vi "Configure.vi"(8 "error in (no error)":errorcluster, 11 "focus in":refnum<class "focus.lvclass">) -> (0 "error out":errorcluster, 2 "cancelled?":bool, 3 "focus out":refnum<class "focus.lvclass">)   [LabVIEW 2012, in "focus.lvclass"]
doc: "The configure method configures the details for the RabbitMQ connection, the observers and the mapping script.\n\nIn the derived class, make a call to the parent for setting these parameters."
uses:
  focus.lvclass
  port_focus.ctl
  baud_rate_focus.ctl
  connection_type_focus.ctl
  <vilib>/Utility/miscctls.llb/LVPointTypeDef.ctl
  focus.lvclass/focus.ctl
  <vilib>/Distrio/Murmex/Murmex/Murmex.lvclass
panel:
  in  "button::ok":bool
  in  "button::configure murmex":bool
  in  "button::cancel":bool
  in  "Tab Control":enum32{"COM ", "Debug"}(tab)
  in  "Port":T1 items=["COM1", "COM2", "COM3", "COM4", "COM5", "COM6", "COM7", "COM8", "COM9", "COM10", "COM11", "COM12", "COM13", "COM14", "COM15", "COM16", "COM17", "COM18", "COM19", "COM20", "COM21", "COM22", "COM23", "COM24", "COM25", "COM26", "COM27", "COM28", "COM29", "COM30"]
  in  "Baudrate":T2=3 items=["9600", "14400", "19200", "38400", "57600", "115200"]
  in  "update frequency":dbl[unit]
  in  "soft limit min":dbl
  in  "soft limit max":dbl
  in  "S/N Master controller":string
  in  "Interface":T3=enum."USB_DaisyChain"
  in  "startup speed":dbl[unit]
  # "RabbitMQ parameters"
  # "Window position"
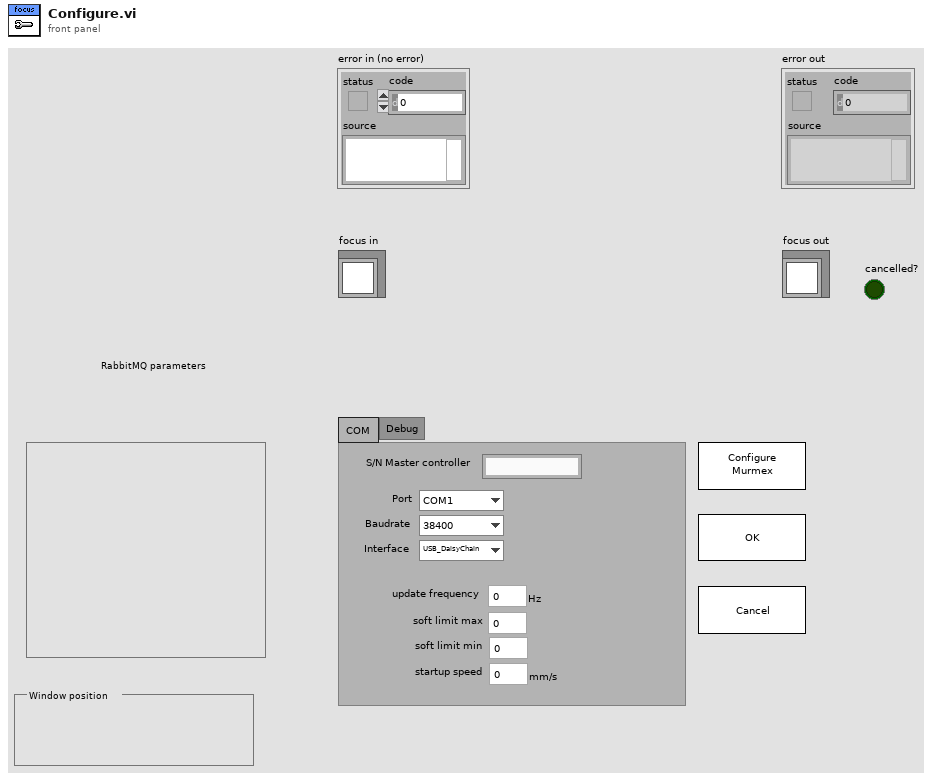
[diagram p1: front panel]
types:
  T1 = typedef "focus.lvclass/port_focus.ctl" = i32
  T2 = typedef "focus.lvclass/baud_rate_focus.ctl" = u16
  T3 = typedef "focus.lvclass/connection_type_focus.ctl" = enum16{"RS232", "RS232 DaisyChain", "USB", "USB_DaisyChain"}
  T4 = typedef "LVPointTypeDef.ctl" = cluster{"Horizontal":i16, "Vertical":i16}
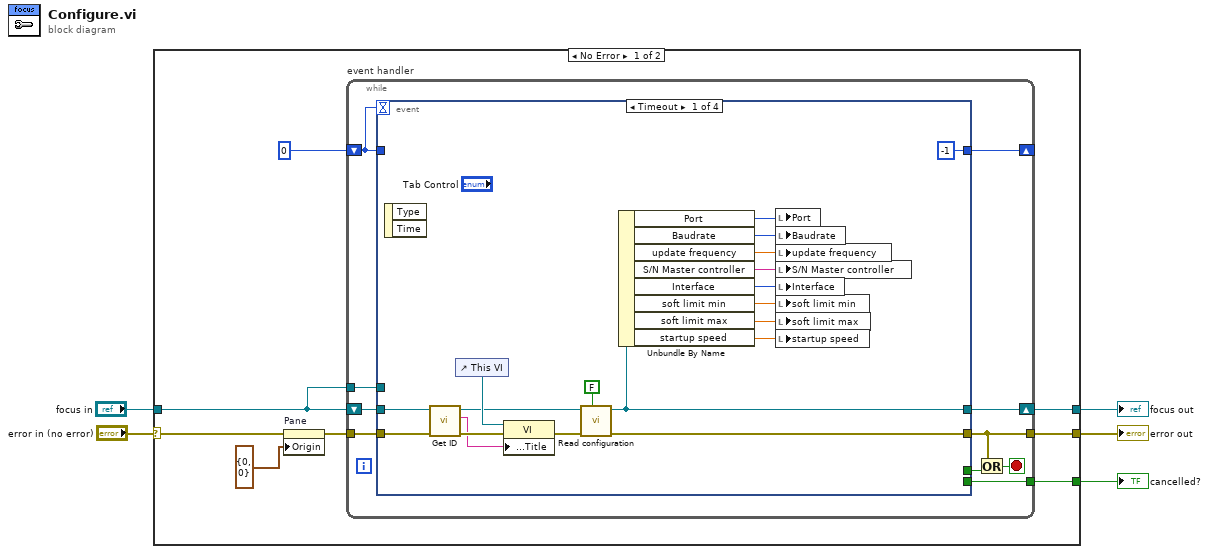
[diagram p0: block diagram]
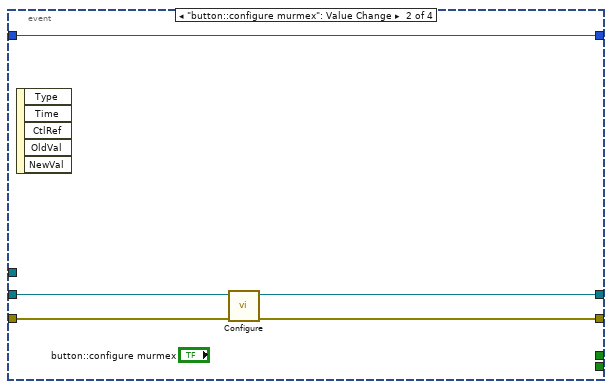
[diagram p2: hidden frame]
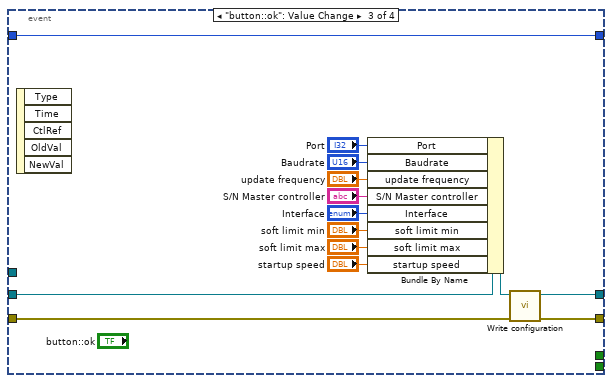
[diagram p3: hidden frame]
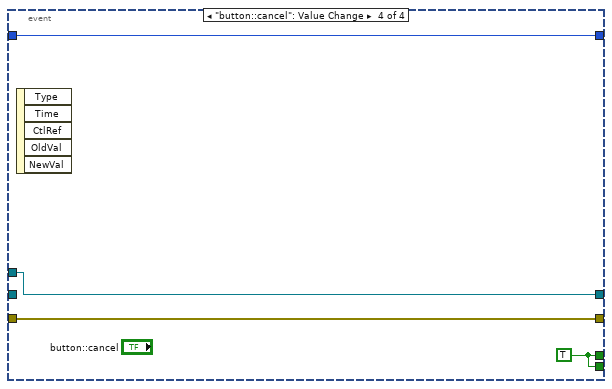
[diagram p4: hidden frame]
diagram:
  n1 = case shown="No Error" "error in (no error)" {
    selector: "error in (no error)" -> [w12 w67]
    tunnel: "focus in" -> [w10 w66]
    tunnel: [w8 w67] -> w3
    tunnel: [w7 w66] -> w2
    tunnel: [w6 _] -> w1
    frame No Error {
      n2 = property on="Pane" class="Pane"(error in=w12, "Origin"=T4 {"Horizontal"=0, "Vertical"=0}) -> (error out=w9:errorcluster)  [unwired: 1 in, 1 out]
      n3 = while "event handler" {
        shift-right: [w22] -> _
        shift-left: 0 -> [w23]
        shift-right: [w18] -> w7
        shift-left: w10 -> [w20]
        tunnel: w10 -> [w21]
        tunnel: w9 -> [w19]
        tunnel: [w16] -> w8
        tunnel: [w14] -> w6
        stop <- w17 stop-if-true
        n4 = event shown="[0] Timeout" {
          selector: _ -> [_ _ _ _]
          dyn-events: _ -> [_ _ _ _]
          timeout: w23 -> [_ _ _ _]
          tunnel: w23 -> [_ w43 w48 w63]
          tunnel: [-1 w43 w48 w63] -> w22
          tunnel: w21 -> [_ _ _ w64]
          tunnel: w20 -> [w39 w45 w58 _]
          tunnel: w19 -> [w42 w47 w61 w65]
          tunnel: [w35 w44 w59 w64] -> w18
          tunnel: [w34 w46 w60 w65] -> w16
          tunnel: [_ _ _ w62] -> w15
          tunnel: [_ _ _ w62] -> w14
          event Timeout {
            n5 = event-data() -> ()  [unwired: 1 in, 2 out]
            n6 = call <vilib>:"Get ID.vi"("error in (no error)"=w42, "Murmex in"=w39) -> ("error out"=w41:errorcluster, "component id"=w24:string, "Murmex out"=w36:refnum<class "focus.lvclass">)  [unwired: 7 in]
            n7 = control-ref of="This VI"() -> (w40:refnum<vi>)
            n8 = property class="VI"(reference=w40, error in=w41, "Front Panel.Title"=w24) -> (error out=w38:errorcluster)  [unwired: 1 out]
            n9 = call-dynamic "Read configuration.vi"("force loading?"=FALSE, "error in (no error)"=w38, "focus in"=w36) -> ("error out"=w34:errorcluster, "focus out"=w35:refnum<class "focus.lvclass">)  [unwired: 7 in]
            n10 = Unbundle By Name(w35) -> ("Port"=w32:T1, "Baudrate"=w31:T2, "update frequency"=w30:dbl[unit], "S/N Master controller"=w29:string, "Interface"=w28:T3, "soft limit min"=w27:dbl, "soft limit max"=w26:dbl, "startup speed"=w25:dbl[unit])
            n11 = local write "Port"(w32) -> ()
            n12 = local write "Baudrate"(w31) -> ()
            n13 = local write "update frequency"(w30) -> ()
            n14 = local write "S/N Master controller"(w29) -> ()
            n15 = local write "Interface"(w28) -> ()
            n16 = local write "soft limit min"(w27) -> ()
            n17 = local write "soft limit max"(w26) -> ()
            n18 = local write "startup speed"(w25) -> ()
          }
          event "button::configure murmex": Value Change {
            n19 = event-data() -> ()  [unwired: 1 in, 5 out]
            n20 = call-parent "Configure.vi"("error in (no error)"=w47, "Murmex in"=w45) -> ("error out"=w46:errorcluster, "Murmex out"=w44:refnum<class "focus.lvclass">)  [unwired: 7 in, 1 out]
          }
          event "button::ok": Value Change {
            n21 = event-data() -> ()  [unwired: 1 in, 5 out]
            n22 = Bundle By Name(cluster=w58, "Port"="Port", "Baudrate"="Baudrate", "update frequency"="update frequency", "S/N Master controller"="S/N Master controller", "Interface"="Interface", "soft limit min"="soft limit min", "soft limit max"="soft limit max", "startup speed"="startup speed") -> (w57:refnum<class "focus.lvclass">)
            n23 = call-dynamic "Write configuration.vi"("error in (no error)"=w61, "focus in"=w57) -> ("error out"=w60:errorcluster, "focus out"=w59:refnum<class "focus.lvclass">)  [unwired: 8 in]
          }
          event "button::cancel": Value Change {
            w62 = TRUE
            n24 = event-data() -> ()  [unwired: 1 in, 5 out]
          }
        }
        n25 = Or(x=w16, y=w15) -> (x .or. y?=w17:bool)
      }
    }
    frame Error {
    }
  }
  "error out" <- w3
  "focus out" <- w2
  "cancelled?" <- w1
